vi "Y calculator.vi"(9 "Blue":u16, 10 "Green":u16, 11 "Red":u16) -> (3 "Y":dbl)   [LabVIEW 2014, in "AMS TS3472 Light Sensor.lvlib" / "AMS TCS3472.lvclass"]
uses:
  AMS TCS3472.lvclass
panel:
  out "x*y 3":dbl
  out "x*y 2":dbl
  out "x*y":dbl
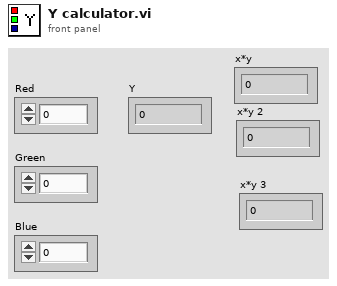
[diagram p1: front panel]
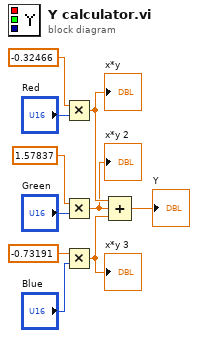
[diagram p0: block diagram]
diagram:
  n1 = Multiply(x=-0.32466, y="Red") -> (x*y=w7:dbl)
  "x*y" <- w7
  n2 = Multiply(x=1.57837, y="Green") -> (x*y=w6:dbl)
  "x*y 2" <- w6
  n3 = Multiply(x=-0.73191, y="Blue") -> (x*y=w5:dbl)
  "x*y 3" <- w5
  n4 = Compound Arithmetic op=ADD(w7, w6, w5) -> (→"Y":dbl)
